vi "Write Reference Mode.vi"(10 "Reference Mode":enum16{"Internal", "External"}(ring), 11 "Signal Generator in":refnum<class "Signal Generator.lvclass">) -> (3 "Signal Generator out":refnum<class "Signal Generator.lvclass">)   [LabVIEW 2020, in "Signal Generator.lvclass"]
uses:
  Signal Generator.lvclass
  Signal Generator.lvclass/Signal Generator.ctl
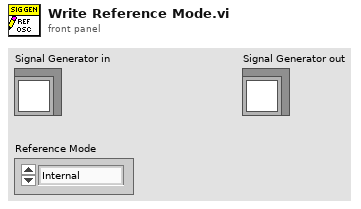
[diagram p1: front panel]
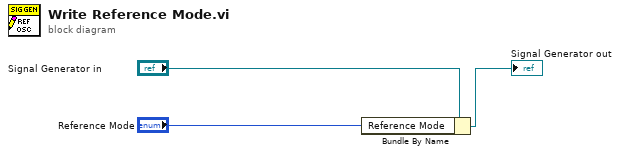
[diagram p0: block diagram]
diagram:
  n1 = Bundle By Name(cluster="Signal Generator in", "Reference Mode"="Reference Mode") -> (→"Signal Generator out":refnum<class "Signal Generator.lvclass">)
